vi "发送失败数据记录到临时文档.vi"(7 "错误输入":errorcluster, 10 "数组":string[](array[string])) -> (0 "错误输出":errorcluster)   [LabVIEW 2016, in "数据传输系统-05.lvlib"]
uses:
  <vilib>/Utility/sysdir.llb/System Directory Type.ctl
panel:
  out "路径":path
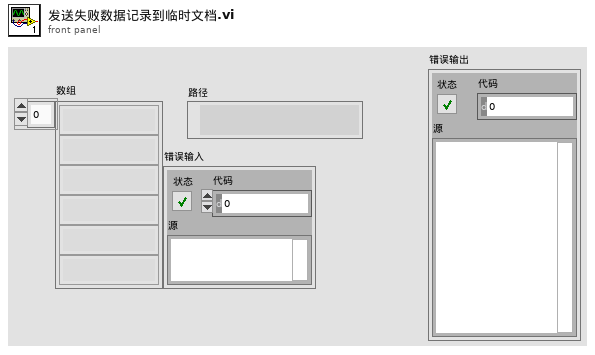
[diagram p1: front panel]
types:
  T1 = typedef "System Directory Type.ctl" = i32
  T2 = enum16{"open", "replace", "create", "open or create", "replace or create", "replace or create with confirmation"}
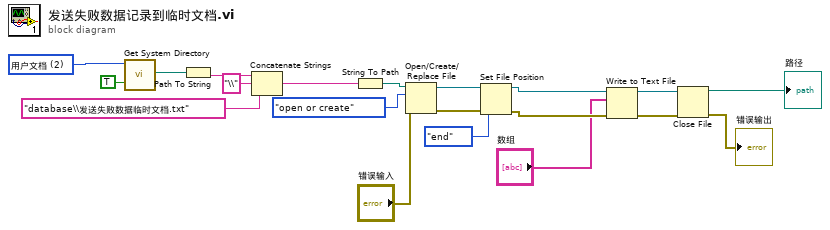
[diagram p0: block diagram]
diagram:
  w13 = T1 2 items=["用户目录"=0, "用户桌面"=1, "用户文档"=2, "用户应用程序数据"=3, "用户设置"=4, "用户临时目录"=5, "公共文档"=6, "公共应用程序数据"=7, "公共设置"=8, "公共缓存"=13, "系统核心库"=9, "系统安装库"=10, "应用程序文件"=11, "启动盘根目录"=12] ("system directory type")
  n1 = call <vilib>:"Get System Directory.vi"("create directory if not found? (F)"=TRUE, "system directory type"=w13) -> ("system directory"=w11:path)  [unwired: 9 in]
  n2 = Path To String(path=w11) -> (string=w10:string)
  n3 = Concatenate Strings(w10, "\\" ("字符串"), "database\\发送失败数据临时文档.txt" ("字符串")) -> (w7:string)
  n4 = String To Path(string=w7) -> (path=w16:path)
  n5 = Open/Create/Replace File(file path (use dialog)=w16, error in="错误输入", operation (0:open)=T2."open or create" ("操作(0:open)")) -> (refnum out=w6:refnum<file>, error out=w5:errorcluster)  [unwired: 3 in, 1 out]
  n6 = Set File Position(refnum=w6, from (0:start)=enum16{"start", "end", "current"}."end" ("自（0:起始）"), error in=w5) -> (refnum out=w4:refnum<file>, error out=w3:errorcluster)  [unwired: 1 in]
  n7 = Write to Text File(file (use dialog)=w4, text="数组", error in=w3) -> (refnum out=w19:refnum<file>, error out=w20:errorcluster)  [unwired: 1 in, 1 out]
  n8 = Close File(refnum=w19, error in=w20) -> (path=→"路径":path, error out=→"错误输出":errorcluster)
